vi "VCH_GEN - Para Management FGV.vi"(8 "error in":errorcluster) -> (0 "error out":errorcluster)   [LabVIEW 2016]
uses:
  Ctrls/VCH _ Parameters.ctl
panel:
  in  "VCH Para":T1
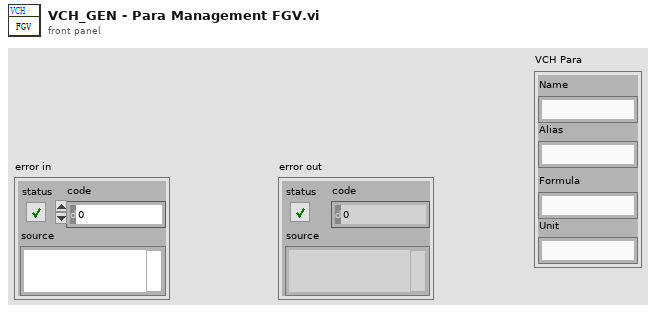
[diagram p1: front panel]
types:
  T1 = typedef "VCH _ Parameters.ctl" = cluster{"Name":string, "Alias":string, "Formula":string, "Unit":string}
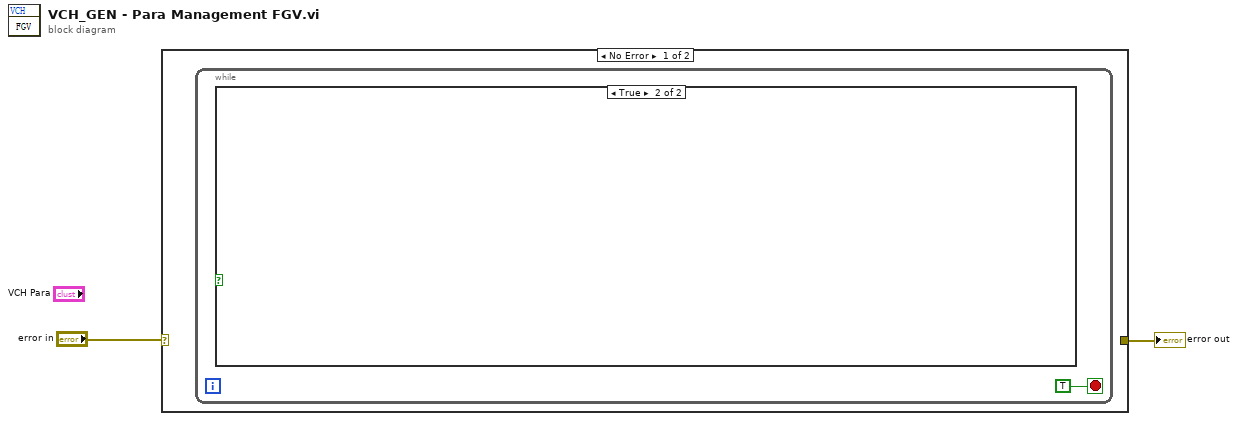
[diagram p0: block diagram]
diagram:
  n1 = case shown="No Error" "error in" {
    selector: "error in" -> [_ w4]
    tunnel: [_ w4] -> w1
    frame No Error {
      n2 = while {
        stop <- TRUE stop-if-true
        n3 = case shown="True" {
          selector: _ -> [_ _]
          frame False {
          }
          frame True {
          }
        }
      }
    }
    frame Error {
    }
  }
  "error out" <- w1
